vi "Configure Reference Level.vi"(8 "error in (no error)":errorcluster, 10 "Reference Level [dBm]":dbl, 11 "MXA in":refnum<class "MXA.lvclass">) -> (0 "error out":errorcluster, 3 "MXA out":refnum<class "MXA.lvclass">)   [LabVIEW 2020, in "MXA.lvclass"]
uses:
  MXA.lvclass
  C:/Sandbox/RF Bench/Source Code/WiSpry Test Framework/Instruments/Spectrum Analyzer/Spectrum Analyzer.lvclass
  C:/Sandbox/RF Bench/Source Code/WiSpry Test Framework/Instruments/Instrument.lvclass
  Instrument.lvclass/Instrument.ctl
  Spectrum Analyzer.lvclass/Spectrum Analyzer.ctl
  <instrlib>/Agilent MXA Series/Public/Configure/Configure Level (Normal).vi
  Instrument.lvclass
  <instrlib>/Agilent MXA Series/Agilent MXA Series.lvlib
  Spectrum Analyzer.lvclass
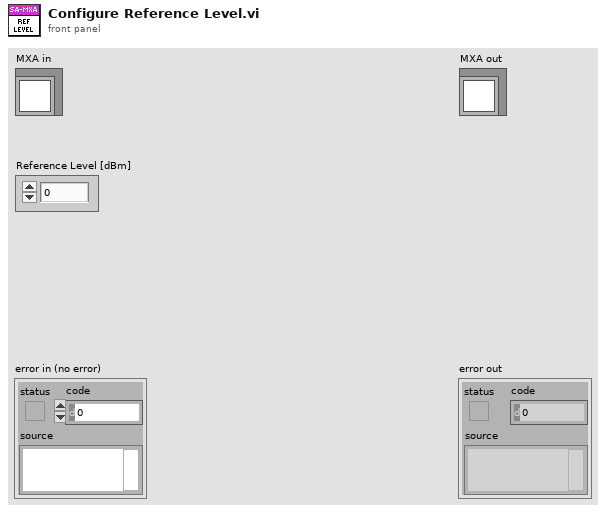
[diagram p1: front panel]
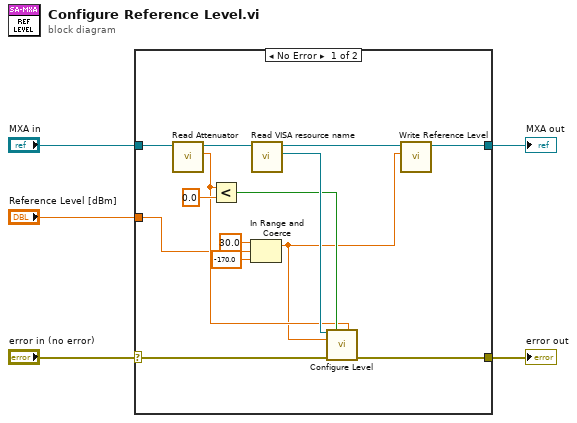
[diagram p0: block diagram]
diagram:
  n1 = case shown="No Error" "error in (no error)" {
    selector: "error in (no error)" -> [w17 w21]
    tunnel: "MXA in" -> [w14 w20]
    tunnel: [w18 w21] -> w5
    tunnel: [w15 w20] -> w4
    tunnel: "Reference Level [dBm]" -> [w9 _]
    frame No Error {
      n2 = call "Read Attenuator.vi"("Spectrum Analyzer in"=w14) -> ("Attenuator"=w10:dbl, "Spectrum Analyzer out"=w13:refnum<class "MXA.lvclass">)  [unwired: 9 in]
      n3 = Less?(x=w10, y=0.0) -> (x < y?=w11:bool)
      n4 = In Range and Coerce(upper limit=30.0, x=w9, lower limit=-170.0) -> (coerced(x)=w6:dbl)  [unwired: 1 out]
      n5 = call "Read VISA resource name.vi"("Instrument in"=w13) -> ("VISA resource name"=w19:refnum<visa-resource-name>, "Instrument out"=w16:refnum<class "MXA.lvclass">)  [unwired: 9 in]
      n6 = call-poly <instrlib>:"Configure Level.vi"("VISA resource name"=w19, "Auto Mechanical Attenuation (T: Enable)"=w11, "Manual Mechanical Attenuation (10 dB)"=w10, "Reference Level (0 dBm)"=w6, "error in (no error)"=w17) -> ("error out"=w18:errorcluster)  [unwired: 9 in, 1 out]
      n7 = call "Write Reference Level.vi"("Reference Level"=w6, "Spectrum Analyzer in"=w16) -> ("Spectrum Analyzer out"=w15:refnum<class "MXA.lvclass">)  [unwired: 9 in]
    }
    frame Error {
    }
  }
  "error out" <- w5
  "MXA out" <- w4
